vi "cRIO_FPGA_COMMUNICATION Global.vi"() -> ()   [LabVIEW 2013, in "cRIO_FPGA_COMMUNICATION.lvlib"]
uses:
  cRIO_FPGA_COMMUNICATION.lvlib
panel:
  out "Stop":bool
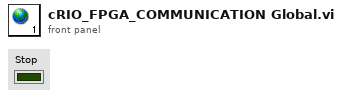
[diagram p1: front panel]
diagram:
